vi "Test Assert Not Equal Value and Type.vi"(8 "error in (no error)":errorcluster) -> (0 "error out":errorcluster)   [LabVIEW 2009]
uses:
  classes/Assert/Assert.lvclass
  classes/Test/Test.lvclass
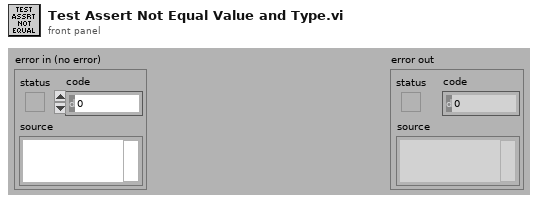
[diagram p1: front panel]
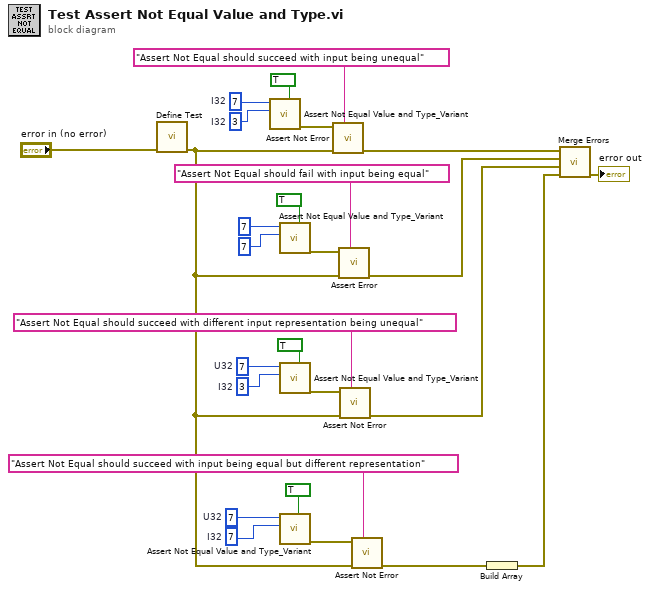
[diagram p0: block diagram]
diagram:
  w7 = 7  # I32
  w8 = u32 7  # U32
  w5 = 3  # I32
  w6 = u32 7  # U32
  w1 = 3  # I32
  w2 = 7  # I32
  n1 = call "Define Test.vi"("error in (no error)"="error in (no error)") -> ("error out"=w19:errorcluster)  [unwired: 10 in]
  n2 = call "Assert Not Equal Value and Type_Variant.vi"("Assert Only? (F)"=TRUE, "Y"=w1, "X"=w2) -> ("error out"=w16:errorcluster)  [unwired: 8 in]
  n3 = call "Assert Not Equal Value and Type_Variant.vi"("Assert Only? (F)"=TRUE, "Y"=7, "X"=7) -> ("error out"=w15:errorcluster)  [unwired: 8 in]
  n4 = call "Assert Not Equal Value and Type_Variant.vi"("Assert Only? (F)"=TRUE, "Y"=w5, "X"=w6) -> ("error out"=w14:errorcluster)  [unwired: 8 in]
  n5 = call "Assert Not Equal Value and Type_Variant.vi"("Assert Only? (F)"=TRUE, "Y"=w7, "X"=w8) -> ("error out"=w12:errorcluster)  [unwired: 8 in]
  n6 = call "Assert Not Error.vi"("Label"="Assert Not Equal should succeed with input being unequal", "error in (no error)"=w19, "Not Error?"=w16) -> ("error out"=w24:errorcluster)  [unwired: 8 in]
  n7 = call "Assert Error.vi"("Label"="Assert Not Equal should fail with input being equal", "error in (no error)"=w19, "Error?"=w15) -> ("error out"=w25:errorcluster)  [unwired: 8 in]
  n8 = call "Assert Not Error.vi"("Label"="Assert Not Equal should succeed with different input representation being unequal", "error in (no error)"=w19, "Not Error?"=w14) -> ("error out"=w21:errorcluster)  [unwired: 8 in]
  n9 = call "Assert Not Error.vi"("Label"="Assert Not Equal should succeed with input being equal but different representation", "error in (no error)"=w19, "Not Error?"=w12) -> ("error out"=w17:errorcluster)  [unwired: 8 in]
  n10 = Build Array(w17) -> (w20:errorcluster[])
  n11 = call <vilib>:"Merge Errors.vi"("error array in"=w20, "error in 3 (no error)"=w21, "error in 2 (no error)"=w25, "error in 1 (no error)"=w24) -> ("error out"=→"error out":errorcluster)  [unwired: 3 in]
